vi "Write SubComponent Raw Data.vi"(5 "Component ID":u8, 7 "FPGA Interface":refnum<class "FPGA Interface.lvclass">, 8 "error in (no error)":errorcluster, 9 "Raw Data":u64[](array[numeric]), 10 "Parameters":string[](array[string]), 11 "1553 SubComponent in":refnum<class "1553 SubComponent.lvclass">) -> (0 "error out":errorcluster)   [LabVIEW 2020, in "BCI-1553 API.lvlib" / "1553 SubComponent.lvclass"]
doc: "Provides a means for taking in a parameter list and raw value and writing it directly to the component in the 1553 Session.\n\nThe parameter is cross-referenced to a memory address and the raw data value is unmodified before being written to the 1553 Session component in bulk."
uses:
  1553 SubComponent.lvclass
  Dependencies/FPGA Interface/FPGA Interface.lvclass
  1553 SubComponent.lvclass/1553 SubComponent.ctl
  Dependencies/Registry/Registry.lvclass/Registry.ctl
  Frames & Messages/TypeDefs/Parameter Table Data.ctl
  Frames & Messages/TypeDefs/Scaling Information.ctl
  Dependencies/Registry/Get Entry.vi
  Dependencies/Registry/Registry.lvclass
  BCI-1553 API.lvlib
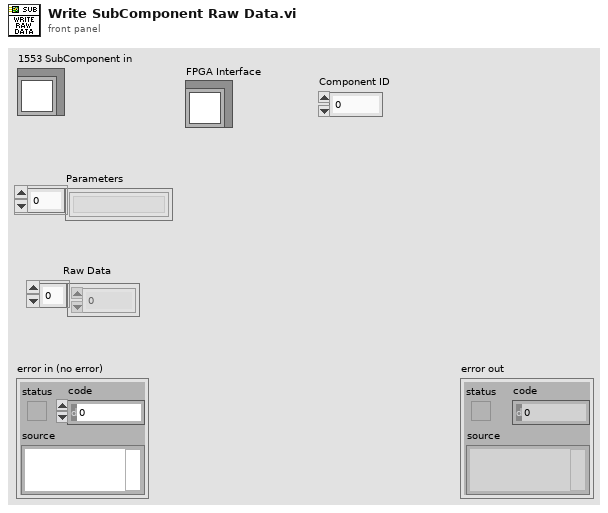
[diagram p1: front panel]
types:
  T1 = typedef "BCI-1553 API.lvlib/Parameter Table Data.ctl" = cluster{"Parameter Name":string, "Base Word":u16, "Address":u16, "Value":u64, "Mask":u16[], "Scaling Info":T2}
  T2 = typedef "BCI-1553 API.lvlib/Scaling Information.ctl" = cluster{"Bit Offset":i32, "Bit Count":i32, "LSB Resolution":dbl, "2's Complement":bool, "Big Endian":bool, "Sign Bit":bool}
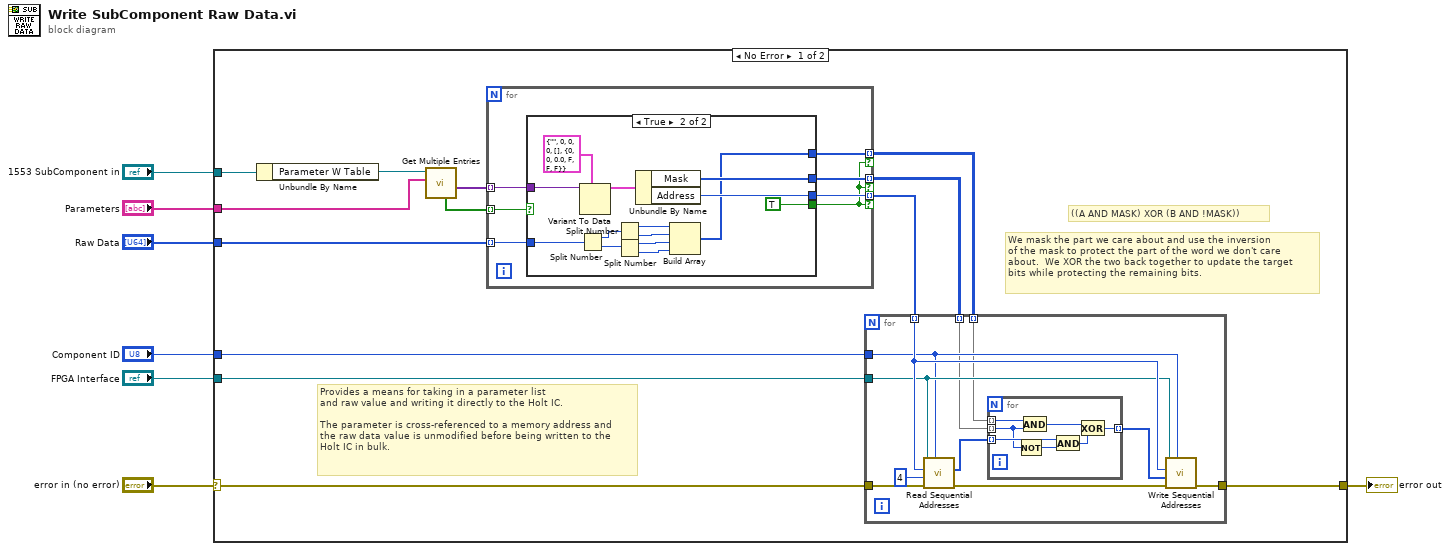
[diagram p0: block diagram]
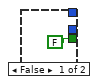
[diagram p2: hidden frame]
diagram:
  n1 = case shown="No Error" "error in (no error)" {
    selector: "error in (no error)" -> [w12 w61]
    tunnel: [w17 w61] -> w1
    tunnel: "1553 SubComponent in" -> [w20 _]
    tunnel: "Parameters" -> [w18 _]
    tunnel: "FPGA Interface" -> [w11 _]
    tunnel: "Component ID" -> [w16 _]
    tunnel: "Raw Data" -> [w13 _]
    frame No Error {
      # "Provides a means for taking in a parameter list\nand raw value and writing it directly to the Holt IC.\n\nThe parameter is cross-referenced to a memory address and\nthe raw data value is unmodified before being written to the\nHolt IC in bulk."
      # "We mask the part we care about and use the inversion\nof the mask to protect the part of the word we don't care\nabout.  We XOR the two back together to update the target\nbits while protecting the remaining bits."
      # "((A AND MASK) XOR (B AND !MASK))"
      n2 = Unbundle By Name(w20) -> ("Parameter W Table"=w19:refnum<class "Registry.lvclass">)
      n3 = call "Get Multiple Entries.vi"("Keys"=w18, "Registry in"=w19) -> ("Values"=w15:variant[], "Found?"=w14:bool[])  [unwired: 6 in, 2 out]
      n4 = for {
        tunnel: w15 -> [w43] mode=indexing
        tunnel: w14 -> [w45] mode=indexing
        tunnel: w13 -> [w44] mode=indexing
        tunnel: [w42] -> w8 mode=indexing if=w39
        tunnel: [w40] -> w10 mode=indexing if=w39
        tunnel: [w41] -> w9 mode=indexing if=w39
        n5 = case shown="True" w45 {
          tunnel: w44 -> [_ w54]
          tunnel: w43 -> [_ w60]
          tunnel: [_ w47] -> w42
          tunnel: [FALSE TRUE] -> w39
          tunnel: [_ w56] -> w41
          tunnel: [_ w55] -> w40
          frame False {
          }
          frame True {
            n6 = Split Number(x=w54) -> (hi(x)=w52:u32, lo(x)=w53:u32)
            n7 = Variant To Data(type=T1 {"Parameter Name"="", "Base Word"=0, "Address"=0, "Value"=0, "Mask"=[], "Scaling Info"={"Bit Offset"=0, "Bit Count"=0, "LSB Resolution"=0.0, "2's Complement"=FALSE, "Big Endian"=FALSE, "Sign Bit"=FALSE}} ("Parameter Table Data"), Variant=w60) -> (data=w58:T1)  [unwired: 1 in, 1 out]
            n8 = Split Number(x=w52) -> (hi(x)=w51:u16, lo(x)=w50:u16)
            n9 = Split Number(x=w53) -> (hi(x)=w49:u16, lo(x)=w48:u16)
            n10 = Unbundle By Name(w58) -> ("Mask"=w56:u16[], "Address"=w55:u16)
            n11 = Build Array(w51, w50, w49, w48) -> (w47:u16[])
          }
        }
      }
      n12 = for {
        tunnel: w16 -> [w25]
        tunnel: w11 -> [w26]
        tunnel: w12 -> [w29]
        tunnel: [w31] -> w17
        tunnel: w9 -> [w23] mode=indexing
        tunnel: w8 -> [w22] mode=indexing
        tunnel: w10 -> [w27] mode=indexing
        n13 = call-dynamic "Read Sequential Addresses.vi"("Target IC (1-8)"=w25, "error in (no error)"=w29, "Addresses to Read"=u16 4, "Starting Address"=w27, "FPGA Interface in"=w26) -> ("error out"=w30:errorcluster, "Data"=w24:u16[])  [unwired: 5 in]
        n14 = for {
          tunnel: w24 -> [w35] mode=indexing
          tunnel: w23 -> [w34] mode=indexing
          tunnel: w22 -> [w33] mode=indexing
          tunnel: [w32] -> w21 mode=indexing
          n15 = Not(x=w34) -> (.not. x?=w37:u16)
          n16 = And(x=w33, y=w34) -> (x .and. y?=w36:u16)
          n17 = And(x=w35, y=w37) -> (x .and. y?=w38:u16)
          n18 = Exclusive Or(1:w38, 2:w36) -> (0:w32:u16)
        }
        n19 = call-dynamic "Write Sequential Addresses.vi"("Target IC (1-8)"=w25, "error in (no error)"=w30, "Data"=w21, "Starting Address"=w27, "FPGA Interface in"=w26) -> ("error out"=w31:errorcluster)  [unwired: 6 in]
      }
    }
    frame Error {
    }
  }
  "error out" <- w1
